vi "Material-Application-MinimumPageSize.vi"(11 "error in":errorcluster) -> (6 "Minimum Pane Size":cluster{"Horizontal":i16, "Vertical":i16}={"Horizontal"=700, "Vertical"=440}, 15 "error out":errorcluster)   [LabVIEW 2013]
panel:
  # "Inputs"
  # "Outputs"
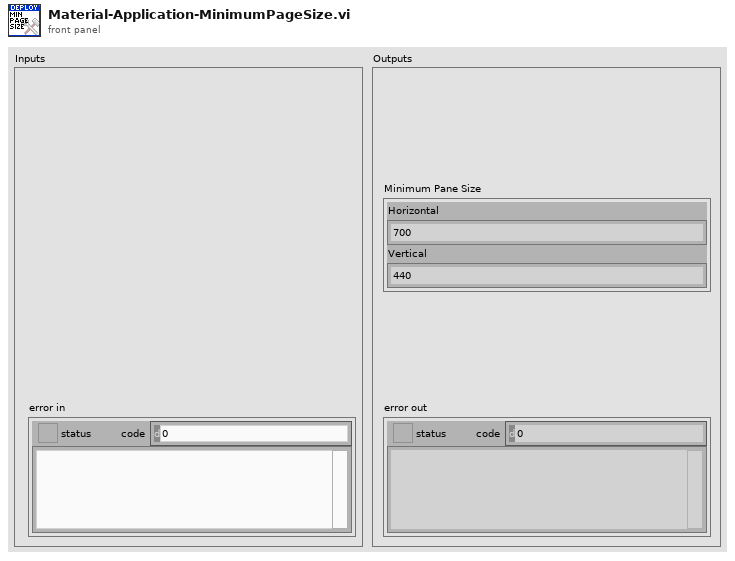
[diagram p1: front panel]
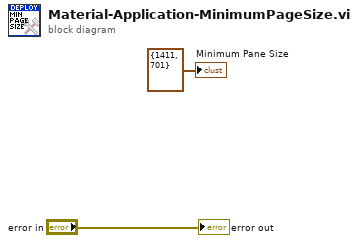
[diagram p0: block diagram]
diagram:
  "error out" <- "error in"
  "Minimum Pane Size" <- cluster{"Horizontal":i16, "Vertical":i16} {"Horizontal"=1411, "Vertical"=701} ("Minimum Pane Size")
